vi "MonitorAccelerometerClock.vi"(11 "Settings":T1={"CommandFIFO"="Accel1CommandFIFO", "SampleTrigger"="Sync/Trig0"}) -> ()   [LabVIEW 2016, in "FPGAMonitorAccelerometer.lvlib"]
uses:
  FPGAMonitorAccelerometer.lvlib
  DataTypes/MonitorAccelerometerClockSettings.ctl
  <vilib>/rvi/Emulation/niFpgaGetClockAttributes.vi
  <vilib>/rvi/Emulation/niFpgaSctlEmulationGetInTimedLoop.vi
  <vilib>/rvi/Emulation/niFpgaEmulationReportErrorSimple.vi
  <vilib>/rvi/DataTransferAndStorage/Container/Common/niFpgaContainerExecOnDevCompGetState.vi
  <vilib>/rvi/Emulation/niFpgaEmulationIsFPGAContextNoSignature.vi
  <vilib>/rvi/errors/niFpgaSetErrorForExecOnDevCompSimple.vi
  <vilib>/rvi/eio/common/nirviEmuReportErrorAndStop.vi
  <vilib>/rvi/DataTransferAndStorage/Container/Common/niFpgaContainerGetUniqueNameForEmu.vi
  <vilib>/rvi/FIFO/Fifo_Resource/nirvififoEmulationSetSize.vi
  <vilib>/rvi/FIFO/Fifo_Resource/nirviFifoEmulationQueueMgr.vi
  <instcachedir>/0/nirviFifoEmulationQueueMgr_E5CAEC123FF24DC58D834DCA3CDAA9B5.lvgen/nirviFifoEmulationQueueMgr_E5CAEC123FF24DC58D834DCA3CDAA9B5_006.vi
  <vilib>/rvi/FIFO/Fifo_Resource/nirvififoEmulationDetermineInputValidOut.vi
  <vilib>/rvi/FIFO/Fifo_Resource/nirvififoEmulationCreateLock.vi
  <vilib>/rvi/Emulation/niFpgaProcessEmulError.vi
  <vilib>/rvi/FIFO/Fifo_Resource/nirvififoEmulationObtainLock.vi
  <vilib>/rvi/FIFO/Fifo_Resource/nirvififoEmulationReleaseLock.vi
  <vilib>/rvi/occurrence/nirviWaitOnOccurrenceBase.vi
  <vilib>/rvi/errors/nirviReportUnexpectedCaseInternalError.vi
  <vilib>/rvi/errors/nirviReportUnexpectedCaseInternalError (U32).vi
  <vilib>/Utility/error.llb/Clear Errors.vi
  <vilib>/rvi/interface/RandomDataEmulation/niFpgaRandomDataHandleErrors.vi
  <vilib>/rvi/eio/common/nirviEmuTemplateMethod_errors.vi
  <vilib>/rvi/Emulation/niFpgaCriticalErrorInLSC.vi
  <vilib>/rvi/DataTransferAndStorage/Container/XNode/niFpgaContainer.xnode
  <vilib>/rvi/FIFO/Fifo_Resource/niFpgaFifoEmulationRefIn.vi
  <vilib>/eio/EIOMethodNode/EIOMethodNode.xnode
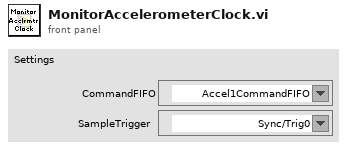
[diagram p1: front panel]
types:
  T1 = typedef "FPGAMonitorAccelerometer.lvlib/MonitorAccelerometerClockSettings.ctl" = cluster{"CommandFIFO":refnum<k21>, "SampleTrigger":refnum<k21>}
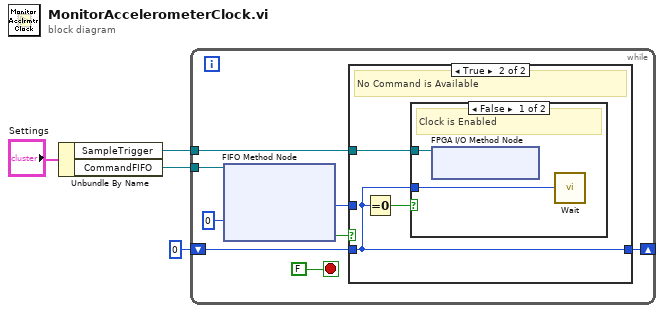
[diagram p0: block diagram]
diagram:
  n1 = Unbundle By Name("Settings") -> ("SampleTrigger"=w1:refnum<k21>, "CommandFIFO"=w2:refnum<k21>)
  n2 = while {
    tunnel: w2 -> [w12]
    shift-right: [w6] -> _
    shift-left: u32 0 -> [w8]
    tunnel: w1 -> [w5]
    stop <- FALSE stop-if-true
    n3 = xnode ("FIFO Method Node")("Timeout"=0, "FIFO In"=w12) -> ("Element"=w9:u32, "Timed Out?"=w10:bool)  [unwired: 1 out]
    n4 = case shown="True" w10 {
      tunnel: w9 -> [w13 _]
      tunnel: w8 -> [_ w14]
      tunnel: [w13 w14] -> w6
      tunnel: w5 -> [_ w15]
      frame False {
        # "A Command is Available"
      }
      frame True {
        # "No Command is Available"
        n5 = Equal To 0?(x=w14) -> (x = 0?=w16:bool)
        n6 = case shown="False" w16 {
          tunnel: w15 -> [w18 _]
          tunnel: w14 -> [w17 _]
          frame False {
            # "Clock is Enabled"
            n7 = xnode "FPGA I/O Method Node"("FPGA I/O In"=w18) -> ()  [unwired: 1 out]
            n8 = call "Wait"("Count(uSec)"=w17) -> ()  [unwired: 1 out]
          }
          frame True {
            # "Clock is Disabled"
          }
        }
      }
    }
  }
